vi "PRIME Detector Get Status.vi"(8 "error in (no error)":errorcluster, 11 "connection ID":refnum<k5>) -> (0 "error out":errorcluster, 1 "Status Response":string, 2 "Status":T1, 3 "connection ID out":refnum<k5>)   [LabVIEW 2021, in "PRIME Detector.lvclass"]
uses:
  PRIME Detector.lvclass
  PRIME Detector cluster Status.ctl
  <vilib>/JDP Science/JSONtext/JSONtext.lvlib
panel:
  out "Status Response 2":string
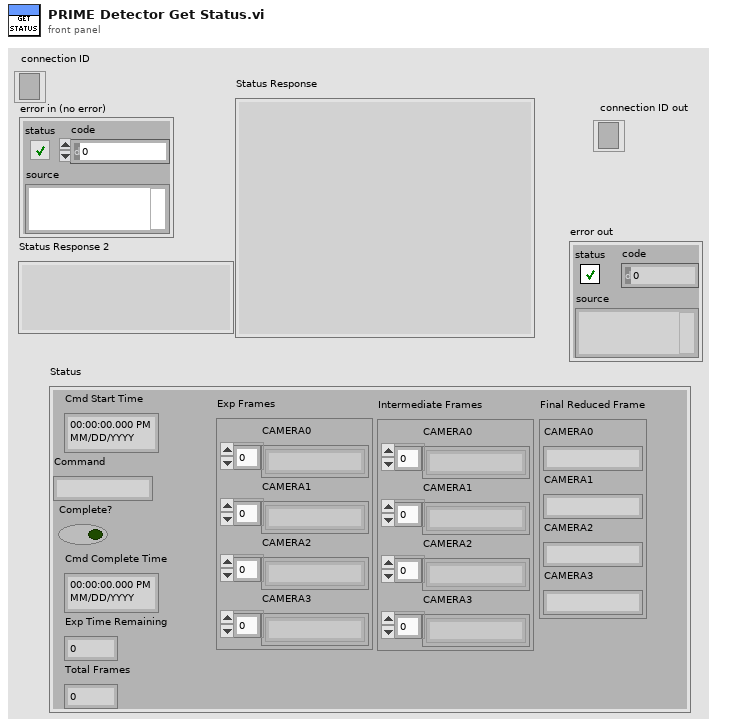
[diagram p1: front panel]
types:
  T1 = typedef "PRIME Detector cluster Status.ctl" = cluster{"Cmd Start Time":timestamp, "Command":string, "Complete?":bool, "Cmd Complete Time":timestamp, "Exp Time Remaining":dbl, "Total Frames":i32, "Exp Frames":cluster{"CAMERA0":string[], "CAMERA1":string[], "CAMERA2":string[], "CAMERA3":string[]}, "Intermediate Frames":cluster{"CAMERA0":string[], "CAMERA1":string[], "CAMERA2":string[], "CAMERA3":string[]}, "Final Reduced Frame":cluster{"CAMERA0":string, "CAMERA1":string, "CAMERA2":string, "CAMERA3":string}}
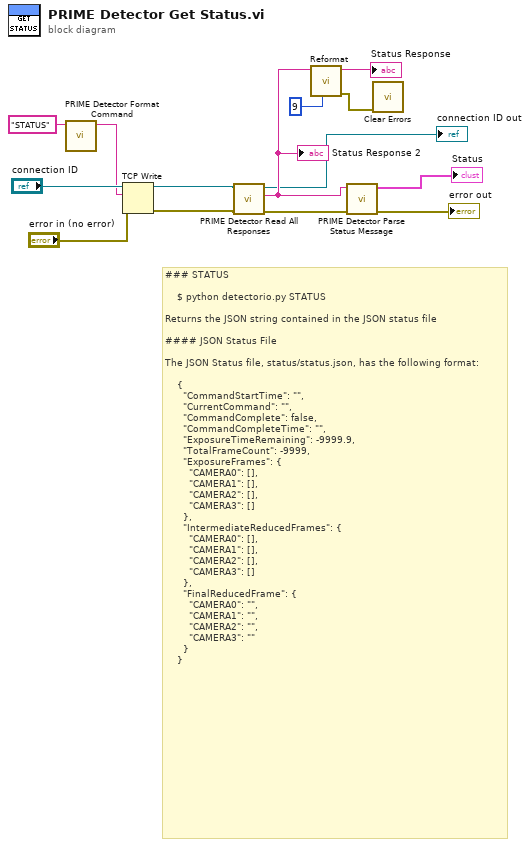
[diagram p0: block diagram]
diagram:
  # "### STATUS\n\n    $ python detectorio.py STATUS\n    \nReturns the JSON string contained in the JSON status file\n\n#### JSON Status File\n\nThe JSON Status file, status/status.json, has the following format:\n\n    {\n      \"CommandStartTime\": \"\",\n      \"CurrentCommand\": \"\",\n      \"CommandComplete\": false,\n      \"CommandCompleteTime\": \"\",\n      \"ExposureTimeRemaining\": -9999.9,\n      \"TotalFrameCount\": -9999,\n      \"ExposureFrames\": {\n        \"CAMERA0\": [],\n        \"CAMERA1\": [],\n        \"CAMERA2\": [],\n        \"CAMERA3\": []\n      },\n      \"IntermediateReducedFrames\": {\n        \"CAMERA0\": [],\n        \"CAMERA1\": [],\n        \"CAMERA2\": [],\n        \"CAMERA3\": []\n      },\n      \"FinalReducedFrame\": {\n        \"CAMERA0\": \"\",\n        \"CAMERA1\": \"\",\n        \"CAMERA2\": \"\",\n        \"CAMERA3\": \"\"\n      }\n    }"
  n1 = call "PRIME Detector Format Command.vi"("Command"="STATUS") -> ("TCP String"=w12:string)  [unwired: 10 in]
  n2 = TCP Write(connection ID="connection ID", data in=w12, error in (no error)="error in (no error)") -> (connection ID out=w10:refnum<k5>, error out=w9:errorcluster)  [unwired: 1 in, 1 out]
  n3 = call "PRIME Detector Read All Responses.vi"("error in"=w9, "connection ID"=w10) -> ("error out"=w7:errorcluster, "Status Response"=w4:string, "connection ID out"=→"connection ID out":refnum<k5>)  [unwired: 6 in, 1 out]
  "Status Response 2" <- w4
  n4 = call <vilib>:"Reformat.vi"("Pretty Print Levels"=9, "JSON"=w4) -> ("error out"=w1:errorcluster, "<JSON>"=→"Status Response":string)  [unwired: 6 in, 2 out]
  n5 = call "PRIME Detector Parse Status Message.vi"("error in (no error)"=w7, "JSON"=w4) -> ("error out"=→"error out":errorcluster, "status"=→"Status":T1)  [unwired: 8 in]
  n6 = call <vilib>:"Clear Errors.vi"("error in (no error)"=w1) -> ()  [unwired: 5 in, 2 out]
